vi "PassiveAggressiveClassifier.vi"(8 "error in":errorcluster) -> (0 "error out":errorcluster, 3 "out":refnum<class "PassiveAggressiveClassifier.lvclass">)   [LabVIEW 2020]
doc: "Available methods:\nGet Attributes\nGet Params\nSet Params"
uses:
  PassiveAggressiveClassifier.lvclass
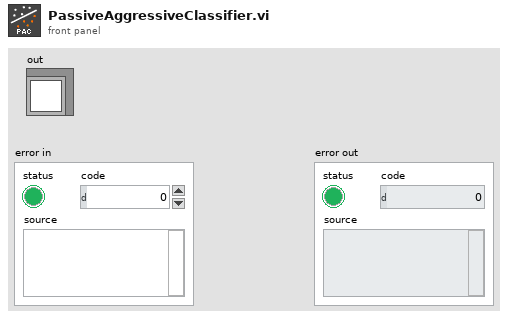
[diagram p1: front panel]
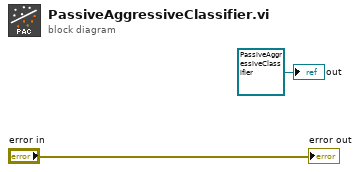
[diagram p0: block diagram]
diagram:
  "out" <- refnum<class "PassiveAggressiveClassifier.lvclass"> refnum ("model")
  "error out" <- "error in"
